vi "Create Timing Channel Array.vi"(10 "incoming channel count (0)":i32, 11 "timing channel ref":T1 format="%.0x") -> (2 "channel offset":i64, 3 "timing channel ref array":T1[](array[typedef]) format="%.0x")   [LabVIEW 2020, in "Ballard MIL-STD-1553 Engine.lvlib" / "Custom Device.lvlib"]
uses:
  Custom Device.lvlib
  <vilib>/NI VeriStand/Custom Device API/Custom Device Item Ref.ctl
  <vilib>/NI VeriStand/Custom Device API/Custom Device API.lvlib
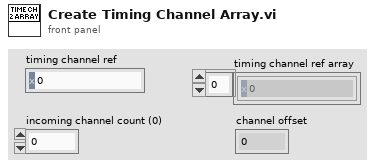
[diagram p1: front panel]
types:
  T1 = typedef "Custom Device API.lvlib/Custom Device Item Ref.ctl" = u64
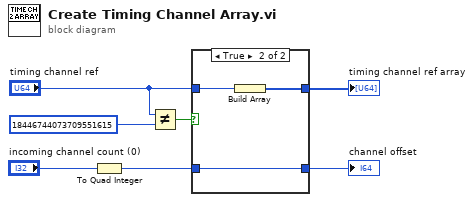
[diagram p0: block diagram]
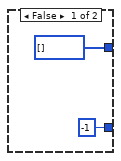
[diagram p2: hidden frame]
diagram:
  n1 = To Quad Integer(1:"incoming channel count (0)") -> (0:w1:i64)
  n2 = Not Equal?(x="timing channel ref", y=T1 18446744073709551615 ("timing channel ref")) -> (x != y?=w6:bool)
  n3 = case shown="True" w6 {
    tunnel: [i64 -1 w10] -> w5
    tunnel: "timing channel ref" -> [_ w12]
    tunnel: [T1[] [] ("s? t:f") w11] -> w3
    tunnel: w1 -> [_ w10]
    frame False {
    }
    frame True {
      n4 = Build Array(w12) -> (w11:T1[])
    }
  }
  "channel offset" <- w5
  "timing channel ref array" <- w3
